vi "writeLogMessage.vi"(8 "error in (no error)":errorcluster, 10 "WriteLogMessageInput":T1, 11 "ITestLog in":refnum<class "ITestLog.lvclass">) -> (0 "error out":errorcluster, 3 "ITestLog out":refnum<class "ITestLog.lvclass">)   [LabVIEW 2015, in "ITestLog.lvclass"]
uses:
  ITestLog.lvclass
  Typedefs/WriteLogMessageInput.ctl
  Typedefs/TestScenarioTypes.ctl
  Typedefs/PassFailTest.ctl
  Typedefs/ILCBTTypedefs.lvlib
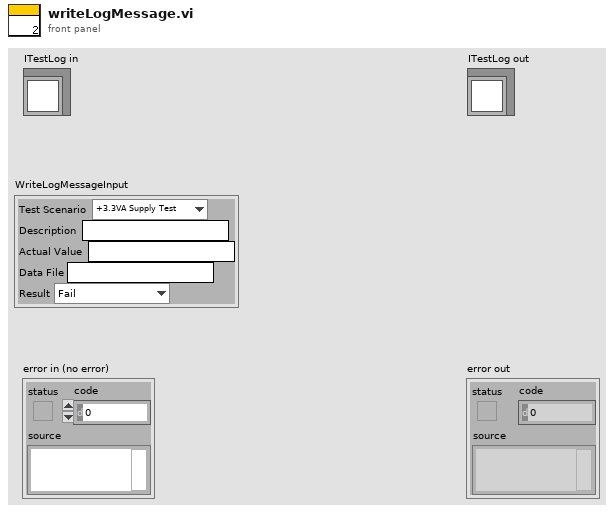
[diagram p1: front panel]
types:
  T1 = typedef "ILCBTTypedefs.lvlib/WriteLogMessageInput.ctl" = cluster{"Test Scenario":T2, "Description":string, "Actual Value":string, "Data File":string, "Result":T3}
  T2 = typedef "ILCBTTypedefs.lvlib/TestScenarioTypes.ctl" = enum16{"+3.3VA Supply Test", "+3.3VD Supply Test", "+5VA Supply Test", "+5VD Supply Test"}
  T3 = typedef "ILCBTTypedefs.lvlib/PassFailTest.ctl" = enum16{"Fail", "Pass", "NA"}
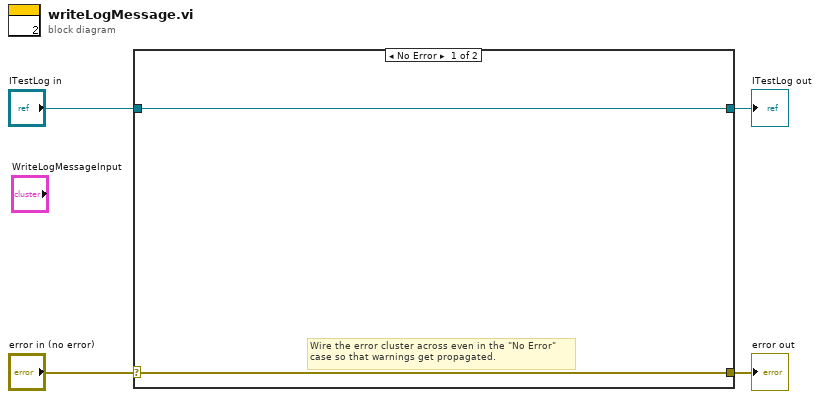
[diagram p0: block diagram]
diagram:
  n1 = case shown="No Error" "error in (no error)" {
    selector: "error in (no error)" -> [w5 w8]
    tunnel: [w5 w8] -> w3
    tunnel: [w6 w7] -> w1
    tunnel: "ITestLog in" -> [w6 w7]
    frame No Error {
      # "Wire the error cluster across even in the \"No Error\"\ncase so that warnings get propagated."
    }
    frame Error {
    }
  }
  "error out" <- w3
  "ITestLog out" <- w1
